vi "SawScan(One axis).vi"() -> ()   [LabVIEW 2012]
uses:
  Madlib.dll
panel:
  in  "Restart Scan Time Delay":u32
  in  "Delay Between Steps (ms)":u32=10
  out "Position (um)":dbl(graph)
  in  "Number of Steps":u16=100 min=1 step=1
  in  "Start  (um)":dbl min=0.0 max=100.0 step=0.5 format="%.3f"
  in  "End  (um)":dbl=100.0 min=0.0 max=100.0 step=0.2 format="%.3f"
  # "This example creates a sawtooth waveform scan in which the nanopositioner moves\nfrom the Start position to the End position following a linear ramp made up of\n\"Number of Steps\" position values with a \"Delay Between Steps\" time spacing.  The\n\"Restart Scan Time Delay\" occurs after a scan is completed and the nanopositioner\nreturns to the Start position."
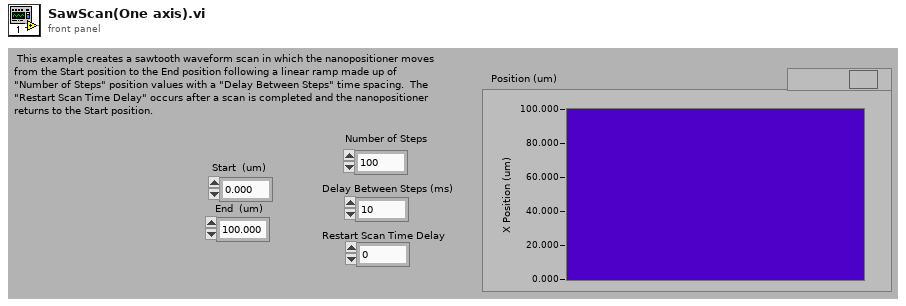
[diagram p1: front panel]
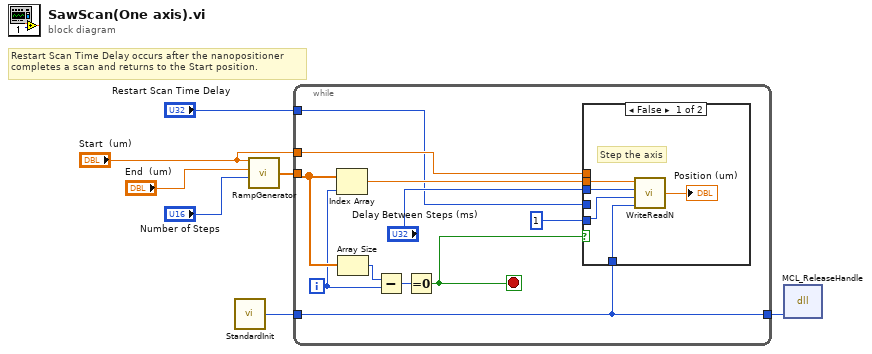
[diagram p0: block diagram]
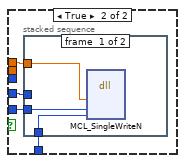
[diagram p2: hidden frame]
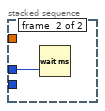
[diagram p3: hidden frame]
diagram:
  # "Restart Scan Time Delay occurs after the nanopositioner\ncompletes a scan and returns to the Start position."
  n1 = call "StandardInit.vi"() -> ("Outgoing Handle"=w1:i32)  [unwired: 1 in]
  n2 = call "RampGenerator.vi"("Number of Positions"="Number of Steps", "End  (um)"="End  (um)", "Start  (um)"="Start  (um)") -> ("Array"=w7:dbl[])  [unwired: 1 in]
  n3 = while {
    tunnel: w7 -> [w16]
    tunnel: "Start  (um)" -> [w11]
    tunnel: "Restart Scan Time Delay" -> [w10]
    tunnel: w1 -> [w9]
    tunnel: [w9] -> w2
    i -> [w14]
    stop <- w15 stop-if-true
    n4 = Index Array(array=w16, index=w14) -> (element=w13:dbl)
    n5 = Array Size(array=w16) -> (size(s)=w17:i32)
    n6 = Subtract(x=w17, y=w14) -> (x-y=w18:i32)
    n7 = Equal To 0?(x=w18) -> (x = 0?=w15:bool)
    n8 = case shown="False" w15 {
      tunnel: w13 -> [w21 _]
      tunnel: "Delay Between Steps (ms)" -> [w22 _]
      tunnel: w11 -> [_ w27]
      tunnel: w10 -> [_ w26]
      tunnel: w9 -> [w20 w25]
      tunnel: 1 -> [w19 w24]
      frame False {
        # "Step the axis"
        n9 = call "WriteReadN.vi"("Handle"=w20, "Axis"=w19, "Delay (ms)"=w22, "Move to (um)"=w21) -> ("Current Position (um)"=→"Position (um)":dbl)
      }
      frame True {
        # "X AXIS SCAN"
        n10 = stacked-sequence {
          tunnel: w27 -> [w30 _]
          tunnel: w26 -> [_ w31]
          tunnel: w25 -> [w29 _]
          tunnel: w24 -> [w28 _]
          frame #0 {
            n11 = dll-call lib="C:/Users/Labview/Desktop/SRR/Madlib_x64/Labview Examples/MADLib.dll" fn="MCL_SingleWriteN"("position"=w30, "axis"=w28, "handle"=w29) -> ()  [unwired: 7 in, 2 out]
          }
          frame #1 {
            n12 = Wait (ms)(milliseconds to wait=w31) -> ()  [unwired: 1 out]
          }
        }
      }
    }
  }
  n13 = dll-call lib="C:/Users/Labview/Desktop/SRR/Madlib_x64/Labview Examples/MADLib.dll" fn="MCL_ReleaseHandle"("handle"=w2) -> ()  [unwired: 5 in, 2 out]
